vi "Fluke Multimeter (No Objects).vi"(8 "error in (no error)":errorcluster, 11 "VISA Resource Name":refnum<visa-resource-name>="GPIB0::2::INSTR") -> (0 "error out":errorcluster, 3 "Fluke Multimeter out":T1)   [LabVIEW 2009]
panel:
  out "Status":string
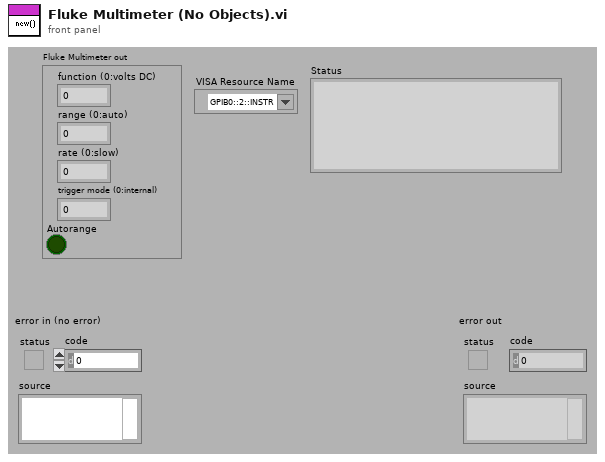
[diagram p1: front panel]
types:
  T1 = cluster{"function (0:volts DC)":u16, "range (0:auto)":u16, "rate (0:slow)":u16, "trigger mode (0:internal)":u16, "Autorange":bool}
  T2 = cluster{"function (0:volts DC)":i16, "range (0:auto)":i16, "rate (0:slow)":i16, "trigger mode (0:internal":i16, "Autorange":bool}
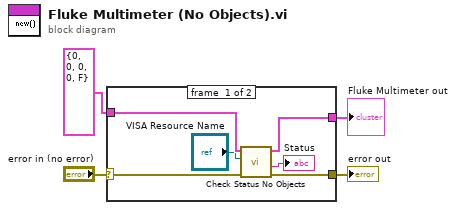
[diagram p0: block diagram]
diagram:
  n1 = case shown="No Error" "error in (no error)" {
    selector: "error in (no error)" -> [w6 w12]
    tunnel: [w9 w12] -> w3
    tunnel: [w10 w11] -> w1
    tunnel: T1 {"function (0:volts DC)"=0, "range (0:auto)"=0, "rate (0:slow)"=0, "trigger mode (0:internal)"=0, "Autorange"=FALSE} ("Initialize Cluster") -> [w7 w11]
    frame #0 {
      n2 = call "Check Status No Objects.vi"("error in (no error)"=w6, "VISA Resource Name"="VISA Resource Name", "input cluster"=w7) -> ("error out"=w9:errorcluster, "Status"=→"Status":string, "output cluster"=w10:T2)  [unwired: 5 in, 1 out]
    }
    frame #1 {
    }
  }
  "error out" <- w3
  "Fluke Multimeter out" <- w1
